vi "BSP2.vi"() -> (1 "핀이 남았다.":bool)   [LabVIEW 2014]
doc: "The myRIO Project template acquires acceleration data from the onboard accelerometer and displays the changes of acceleration values in a waveform chart."
uses:
  <vilib>/vision/driver/NI_Vision_Acquisition_Software.lvlib
  <vilib>/vision/NI_Vision_Development_Module.lvlib
panel:
  out "Number of Particles":i32=6
  in  "Local":T1={"Object Type"=0, "Method"=1, "Niblack Deviation Factor"=1.0, "Window"={"Width"=200, "Height"=200}} {"Niblack Deviation Factor" min=0.0 max=1.0 format="%.2f"; "Method" items=["Niblack", "Background Correction"]; "Object Type" items=["Bright Objects", "Dark Objects"]}
  out "숫자형 컨트롤":i32
  in  "카메라 X":dbl=50.0
  out "볼링핀을찾았는가":bool=TRUE
  out "Image 2":T2(plugin-control)
  out "Image":T2(plugin-control)
  in  "Camera Name":refnum<k21>="cam1" caption="IMAQdx Session"
  # "Control Motor"
  # "Read Encoder"
  # "50"
  # "25"
  # "1일때 + 0일때 -"
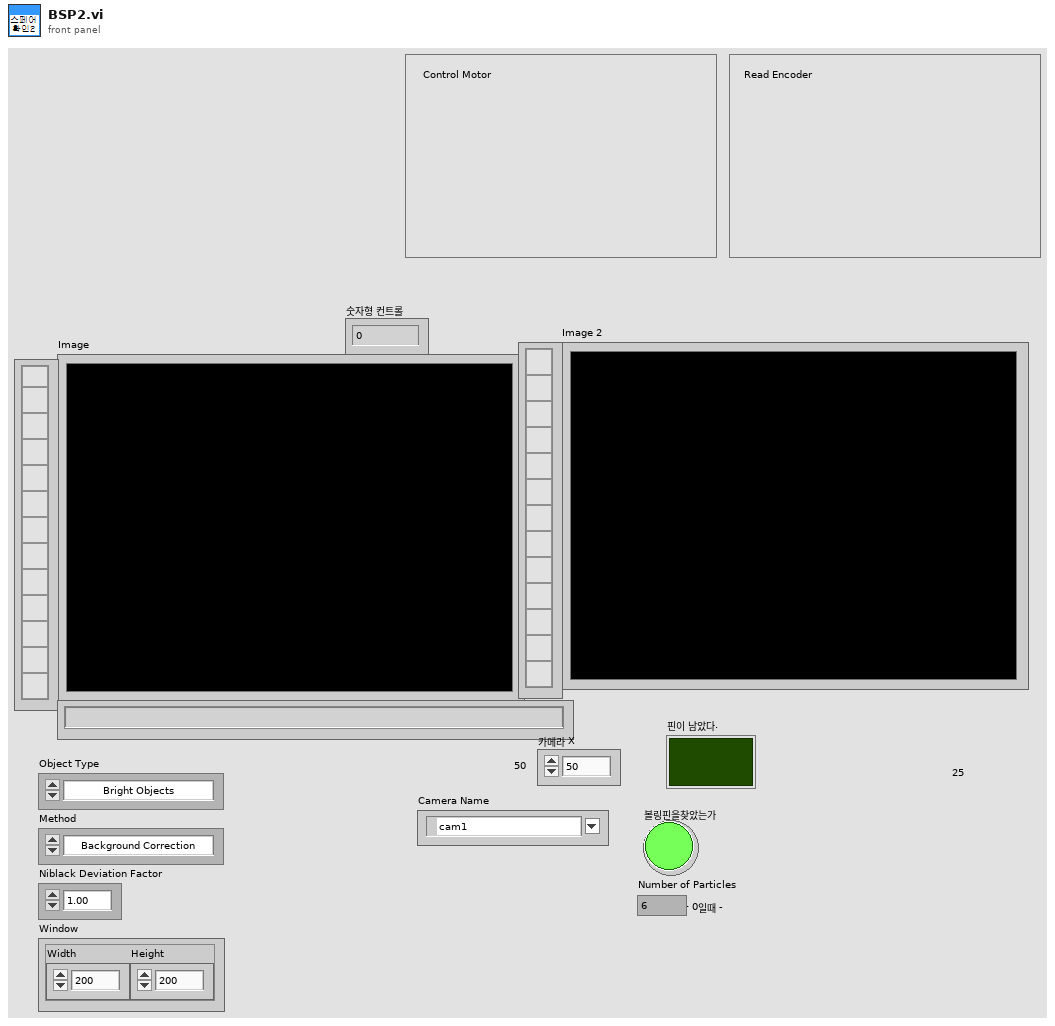
[diagram p1: front panel]
types:
  T1 = cluster{"Object Type":u32, "Method":u32, "Niblack Deviation Factor":dbl, "Window":cluster{"Width":i32, "Height":i32}}
  T2 = typedef "IMAQ Image.ctl" = refnum<image>
  T3 = typedef "IMAQ Rectangle" = cluster{"Left":i32, "Top":i32, "Right":i32, "Bottom":i32, "Rotation":dbl}
  T4 = typedef "IMAQdx.ctl" = refnum<k21>
  T5 = cluster{"Niblack Deviation Factor":dbl, "Niblack Deviation Factor":dbl}
  T6 = cluster{"Global Rectangle":i32[], "Contours":cluster{"Contour Type":u32, "ROI Type":u32, "Points":i32[]}[]}
  T7 = cluster{"Area":dbl, "Number of Holes":dbl, "Bounding Rect":cluster{"Left":dbl, "Top":dbl, "Right":dbl, "Bottom":dbl}, "Center of Mass":cluster{"X":dbl, "Y":dbl}, "Orientation":dbl, "Dimensions":cluster{"Width":dbl, "Height":dbl}}[]
  T8 = cluster{"Left":dbl, "Top":dbl, "Right":dbl, "Bottom":dbl}
  T9 = typedef "ROI Descriptor" = cluster{"Global Rectangle":i32[], "Contours":cluster{"ID":enum32{"External", "Internal"}, "Type":u32, "Coordinates":i32[]}[]}
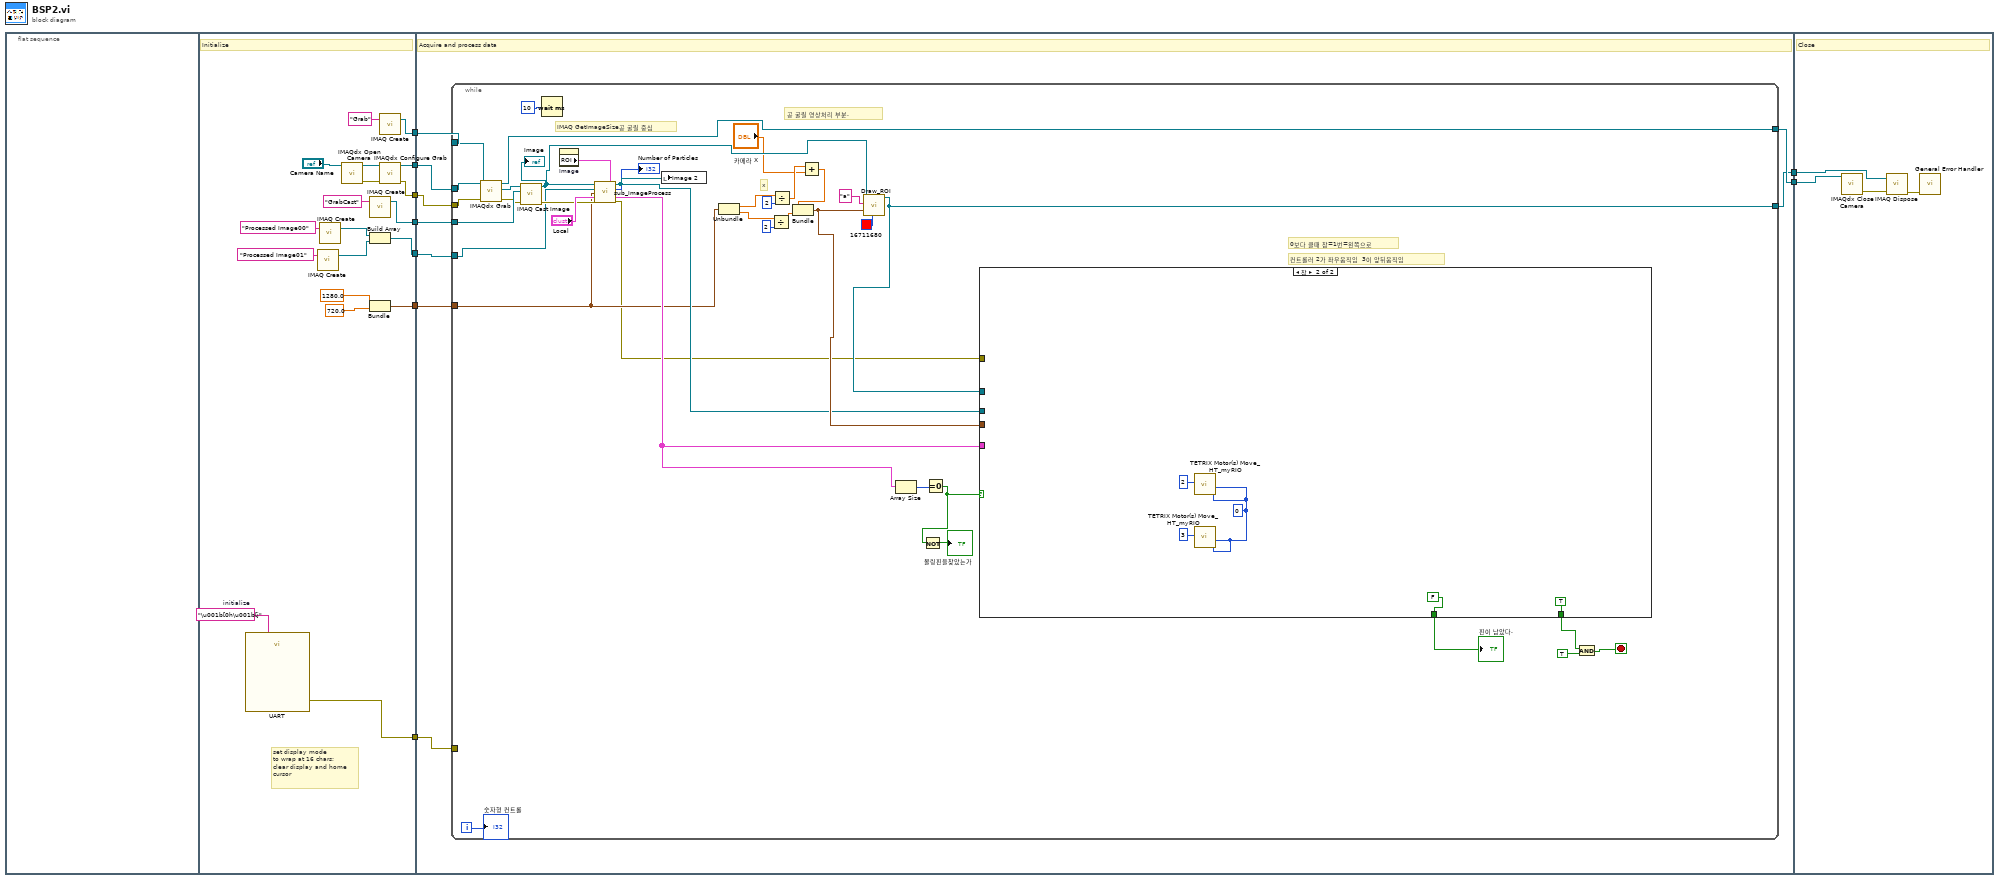
[diagram p0: block diagram]
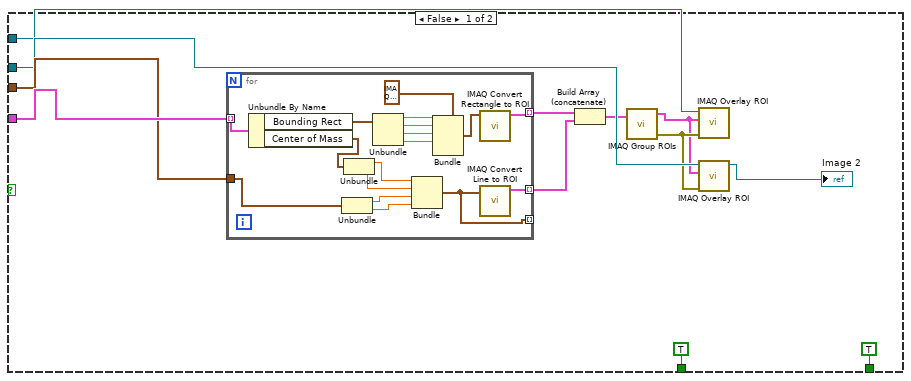
[diagram p2: hidden frame]
diagram:
  n1 = flat-sequence {
    tunnel: [w24] -> w9
    tunnel: [w23] -> w8
    tunnel: [w22] -> w7
    tunnel: [w10] -> w6
    tunnel: [w20] -> w5
    tunnel: [w17] -> w2
    tunnel: [w14] -> w1
    tunnel: w9 -> [w37]
    tunnel: w8 -> [w36]
    tunnel: w7 -> [w35]
    tunnel: [w32] -> w4
    tunnel: [w34] -> w3
    tunnel: w6 -> [w33]
    tunnel: w5 -> [w31]
    tunnel: w2 -> [w30]
    tunnel: w1 -> [w29]
    tunnel: w4 -> [w111]
    tunnel: w3 -> [w110]
    frame #0 {
    }
    frame #1 {
      w19 = "\u001b[0h\u001b[j"  # initialize
      # "set display mode\nto wrap at 16 chars;\nclear display and home\ncursor"
      # "Initialize"
      n2 = call "UART"("Characters to Write"=w19) -> ("error out"=w20:errorcluster)  [unwired: 25 in, 1 out]
      n3 = call "IMAQ Create"("Image Name"="Processed Image01") -> ("New Image"=w11:T2)  [unwired: 3 in, 2 out]
      n4 = call "IMAQ Create"("Image Name"="Processed Image00") -> ("New Image"=w12:T2)  [unwired: 3 in, 2 out]
      n5 = call <vilib>:"IMAQdx Open Camera.vi"("Session In"="Camera Name") -> ("error out"=w28:errorcluster, "Session Out"=w27:T4)  [unwired: 2 in, 7 out]
      n6 = Bundle("Niblack Deviation Factor"=1280.0, "Niblack Deviation Factor"=720.0) -> (w14:T5)  [unwired: 1 in]
      n7 = call "IMAQ Create"("Image Name"="GrabCast") -> ("New Image"=w17:T2)  [unwired: 3 in, 2 out]
      n8 = Build Array(w12, w11) -> (w10:T2[])
      n9 = call "IMAQ Create"("Image Name"="Grab") -> ("New Image"=w24:T2)  [unwired: 3 in, 2 out]
      n10 = call <vilib>:"IMAQdx Configure Grab.vi"("error in"=w28, "Session In"=w27) -> ("error out"=w22:errorcluster, "Session Out"=w23:T4)  [unwired: 8 out]
    }
    frame #2 {
      # "Acquire and process data"
      n11 = while {
        tunnel: [w72] -> w34
        tunnel: w35 -> [w74]
        tunnel: w36 -> [w75]
        tunnel: w37 -> [w73]
        tunnel: w33 -> [w46]
        tunnel: [w63] -> w32
        tunnel: w31 -> [_]
        tunnel: w30 -> [w54]
        tunnel: w29 -> [w45]
        i -> [w51]
        stop <- w57 stop-if-true
        # "공 굴릴 영상처리 부분."
        # "0보다 클때 참=1번=왼쪽으로"
        # "컨트롤러 2가 좌우움직임  3이 앞뒤움직임"
        # "IMAQ GetImageSize공 굴릴 중심"
        # "x"
        n12 = call <vilib>:"IMAQdx Grab.vi"("error in"=w74, "Image In"=w73, "Session In"=w75) -> ("error out"=w53:errorcluster, "Image Out"=w55:T2, "Session Out"=w72:T4)  [unwired: 1 in, 5 out]
        n13 = call "IMAQ Cast Image"("error in (no error)"=w53, "Image Dst"=w54, "Image Src"=w55) -> ("error out"=w49:errorcluster, "Image Dst Out"=w48:T2)  [unwired: 7 in]
        "Image" <- w48
        n14 = Wait (ms)(milliseconds to wait=u32 10 ("대기 시간(ms)")) -> ()  [unwired: 1 out]
        n15 = property on="Image" class="ImageControl"() -> ("ROI"=w52:T6)  [unwired: 2 in, 2 out]
        n16 = call "sub_ImageProcess.vi"("참조 번호 입력"=w48, "ROI"=w52, "배열"=w46, "클러스터"=w45, "Local"="Local", "에러 입력(에러 없음)"=w49) -> ("참조 번호 출력"=w62:T2, "Number of Particles"=→"Number of Particles":i32, "Particle Reports (Pixels)"=w59:T7, "error out"=w42:errorcluster)  [unwired: 6 in]
        n17 = local write "Image 2"(w62) -> ()
        n18 = Unbundle(w45) -> ("Niblack Deviation Factor"=w44:dbl, "Niblack Deviation Factor"=w43:dbl)
        n19 = Divide(x=w43, y=2) -> (x/y=w69:dbl)
        n20 = Divide(x=w44, y=2) -> (x/y=w41:dbl)
        n21 = Add(x=w41, y="카메라 X") -> (x+y=w39:dbl)
        n22 = Bundle(w39, w69) -> (w65:cluster{dbl, dbl})  [unwired: 1 in]
        n23 = call "Draw_ROI.vi"("Color"=u32 16711680, "클러스터"=w65, "Group"="a", "참조 번호 입력"=w48) -> ("참조 번호 출력"=w63:T2)  [unwired: 7 in]
        n24 = Array Size(array=w59) -> (size(s)=w66:i32)
        n25 = Equal To 0?(x=w66) -> (x = 0?=w60:bool)
        n26 = Not(x=w60) -> (.not. x?=→"볼링핀을찾았는가":bool)
        n27 = case shown="참" w60 {
          tunnel: w59 -> [w87 _]
          tunnel: w65 -> [w86 _]
          tunnel: w62 -> [w85 _]
          tunnel: w63 -> [w84 _]
          tunnel: [TRUE TRUE] -> w58
          tunnel: w42 -> [_ _]
          tunnel: [TRUE FALSE] -> w38
          frame False {
            n28 = for {
              tunnel: w87 -> [w104] mode=indexing
              tunnel: [w96] -> w80 mode=indexing
              tunnel: w86 -> [w92]
              tunnel: [w89] -> w82 mode=indexing
              tunnel: [w88] -> _ mode=indexing
              n29 = Unbundle By Name(w104) -> ("Bounding Rect"=w102:T8, "Center of Mass"=w95:cluster{"X":dbl, "Y":dbl})
              n30 = Unbundle(w92) -> (w91:dbl, w90:dbl)
              n31 = Unbundle(w95) -> ("X"=w94:dbl, "Y"=w93:dbl)
              n32 = Unbundle(w102) -> ("Left"=w101:dbl, "Top"=w100:dbl, "Right"=w99:dbl, "Bottom"=w98:dbl)
              n33 = Bundle("X"=w94, "Y"=w93, w91, w90) -> (w88:cluster{"X":dbl, "Y":dbl, dbl, dbl})  [unwired: 1 in]
              n34 = Bundle(cluster=T3 {"Left"=0, "Top"=0, "Right"=0, "Bottom"=0, "Rotation"=0.0} ("Rectangle"), "Left"=w101, "Top"=w100, "Right"=w99, "Bottom"=w98) -> (w97:T3)  [unwired: 1 in]
              n35 = call "IMAQ Convert Rectangle to ROI"("Rectangle"=w97) -> ("ROI Descriptor"=w96:T9)  [unwired: 8 in, 1 out]
              n36 = call "IMAQ Convert Line to ROI"("Line"=w88) -> ("ROI Descriptor"=w89:T9)  [unwired: 8 in, 1 out]
            }
            n37 = Build Array (concatenate)(w80, w82) -> (w81:T9[])
            n38 = call "IMAQ Group ROIs"("ROI Descriptors"=w81) -> ("error out"=w83:errorcluster, "ROI Descriptor out"=w79:T9)  [unwired: 1 in, 2 out]
            n39 = call "IMAQ Overlay ROI"("error in (no error)"=w83, "ROI Descriptor"=w79, "Image"=w84) -> ()  [unwired: 3 in, 6 out]
            n40 = call "IMAQ Overlay ROI"("error in (no error)"=w83, "ROI Descriptor"=w79, "Image"=w85) -> ("Image Out"=→"Image 2":T2)  [unwired: 3 in, 5 out]
          }
          frame True {
            w107 = 0
            n41 = call <vilib>:"TETRIX Motor(s) Move_HT_myRIO.vi"("Motor 2 Power (-100 to 100)\n0 = Stop/Brake\n-128 = Stop/Coast"=w107, "Motor 1 Power (-100 to 100)\n0 = Stop/Brake\n-128 = Stop/Coast"=w107, "Controller Daisy Chain Position: 1 - 4"=u8 2) -> ()  [unwired: 6 in, 1 out]
            n42 = call <vilib>:"TETRIX Motor(s) Move_HT_myRIO.vi"("Motor 2 Power (-100 to 100)\n0 = Stop/Brake\n-128 = Stop/Coast"=w107, "Motor 1 Power (-100 to 100)\n0 = Stop/Brake\n-128 = Stop/Coast"=w107, "Controller Daisy Chain Position: 1 - 4"=u8 3) -> ()  [unwired: 6 in, 1 out]
          }
        }
        "핀이 남았다." <- w38
        n43 = And(x=w58, y=TRUE) -> (x .and. y?=w57:bool)
        "숫자형 컨트롤" <- w51
      }
    }
    frame #3 {
      # "Close"
      n44 = call <vilib>:"IMAQdx Close Camera.vi"("Session In"=w110) -> ("error out"=w113:errorcluster)  [unwired: 1 in, 9 out]
      n45 = call "IMAQ Dispose"("Image"=w111, "error in (no error)"=w113) -> ("error out"=w112:errorcluster)  [unwired: 4 in]
      n46 = call <vilib>:"General Error Handler.vi"("error in (no error)"=w112) -> ()  [unwired: 2 in, 13 out]
    }
  }
